vi "write_attributes.vi"(8 "error in (no error)":errorcluster, 10 "attributes":T1, 11 "MeanShift in":refnum<class "MeanShift.lvclass">) -> (0 "error out":errorcluster, 3 "MeanShift out":refnum<class "MeanShift.lvclass">)   [LabVIEW 2020, in "MeanShift.lvclass"]
uses:
  MeanShift.lvclass
  Controls/mean_shift_attributes.ctl
  MeanShift.lvclass/MeanShift.ctl
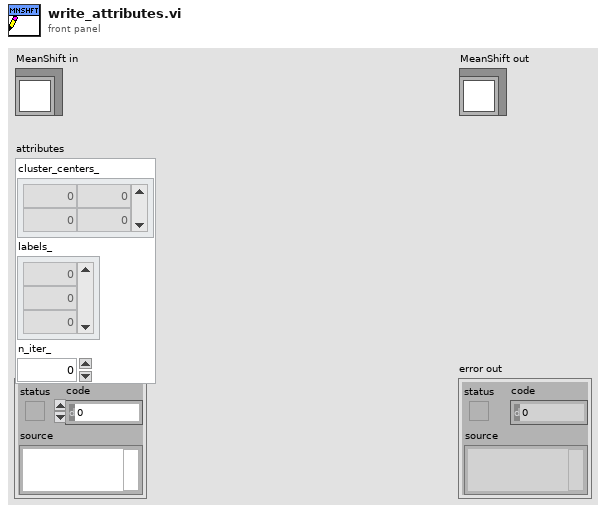
[diagram p1: front panel]
types:
  T1 = typedef "mean_shift_attributes.ctl" = cluster{"cluster_centers_":dbl[][], "labels_":dbl[], "n_iter_":dbl}
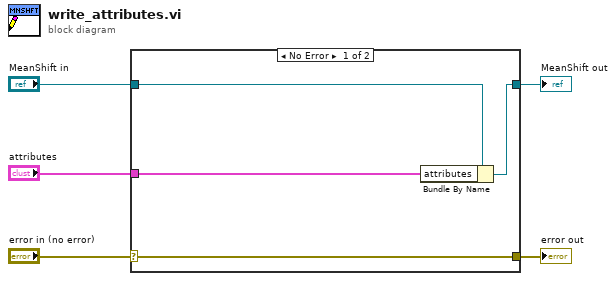
[diagram p0: block diagram]
diagram:
  n1 = case shown="No Error" "error in (no error)" {
    selector: "error in (no error)" -> [w9 w10]
    tunnel: [w9 w10] -> w4
    tunnel: [w7 w11] -> w2
    tunnel: "MeanShift in" -> [w8 w11]
    tunnel: "attributes" -> [w6 _]
    frame No Error {
      n2 = Bundle By Name(cluster=w8, "attributes"=w6) -> (w7:refnum<class "MeanShift.lvclass">)
    }
    frame Error {
    }
  }
  "error out" <- w4
  "MeanShift out" <- w2
